vi "GetErrors.vi"(8 "error in (no error)":errorcluster, 11 "reference in":refnum<class "MLA.lvclass">) -> (0 "error out":errorcluster, 1 "Errors since last call":string, 2 "New Errors":bool, 3 "reference out":refnum<class "MLA.lvclass">, 4 "Errors since last clear":string, 5 "Uncleared Errors":bool)   [LabVIEW 2017, in "MLA.lvclass"]
uses:
  MLA.lvclass
  S5Tools/ErrorLog/ErrorLog.lvclass
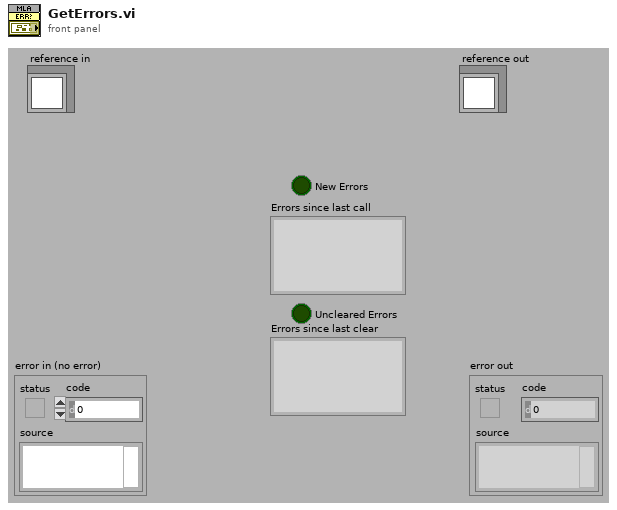
[diagram p1: front panel]
types:
  T1 = typedef "MLA.lvclass/ObjectAttributes.ctl" = cluster{"App Name":string, "App Version":string, "Revision History":string, "Log File Path":path, "Config INI File":path, "Config Path":path, "Log Archive Path":path, "Msg Q's":refnum<queue>[], "VI":refnum<vi>, "ErrLog":refnum<class "ErrorLog.lvclass">}
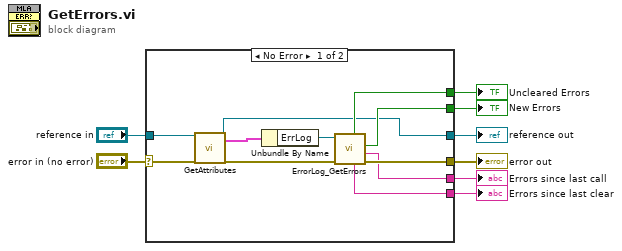
[diagram p0: block diagram]
diagram:
  n1 = case shown="No Error" "error in (no error)" {
    selector: "error in (no error)" -> [w19 w21]
    tunnel: [w15 w21] -> w7
    tunnel: [w9 w20] -> w5
    tunnel: "reference in" -> [w18 w20]
    tunnel: [w13 _] -> w4
    tunnel: [w12 _] -> w3
    tunnel: [w11 _] -> w2
    tunnel: [w10 _] -> w1
    frame No Error {
      n2 = call "GetAttributes.vi"("MLA"=w18, "error in (no error)"=w19) -> ("MLA"=w9:refnum<class "MLA.lvclass">, "Data"=w16:T1, "error out"=w17:errorcluster)  [unwired: 14 in, 1 out]
      n3 = Unbundle By Name(w16) -> ("ErrLog"=w14:refnum<class "ErrorLog.lvclass">)
      n4 = call-dynamic "ErrorLog_GetErrors.vi"("error in (no error)"=w17, "reference in"=w14) -> ("error out"=w15:errorcluster, "Errors since last call"=w10:string, "New Errors"=w12:bool, "Errors since last clear"=w11:string, "Uncleared Errors"=w13:bool)  [unwired: 4 in, 1 out]
    }
    frame Error {
    }
  }
  "error out" <- w7
  "reference out" <- w5
  "Errors since last call" <- w1
  "New Errors" <- w3
  "Errors since last clear" <- w2
  "Uncleared Errors" <- w4
